vi "FlpLib ABCtoDQ_noSine_3PhasePowInv 4.vi"(0 "A":sgl, 1 "cosx":sgl, 2 "sinx":sgl, 5 "B":sgl, 7 "C":sgl) -> (4 "direct":sgl, 6 "quadrature":sgl, 10 "alpha":sgl, 15 "beta":sgl)   [LabVIEW 2017]
uses:
  ABCtoAlphaBeta_3PhasePowInv/FlpLib ABCtoAlphaBeta_3PhasePowInv 4.vi
  AlphaBetaToDQ_noSine/FlpLib AlphaBetaToDQ_noSine 4.vi
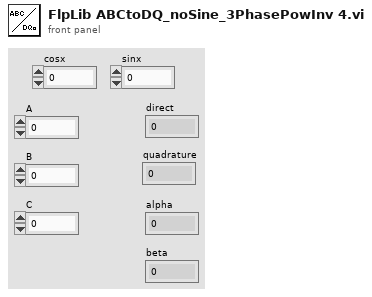
[diagram p1: front panel]
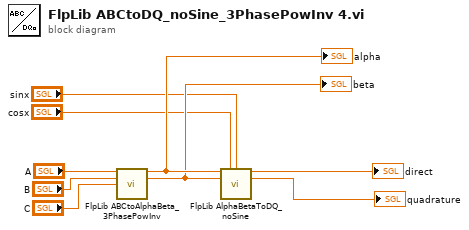
[diagram p0: block diagram]
diagram:
  n1 = call-poly "FlpLib ABCtoAlphaBeta_3PhasePowInv.vi"("A"="A", "B"="B", "C"="C") -> ("alpha"=w9:sgl, "beta"=w8:sgl)  [unwired: 11 in]
  "alpha" <- w9
  "beta" <- w8
  n2 = call-poly "FlpLib AlphaBetaToDQ_noSine.vi"("alpha"=w9, "cosx"="cosx", "sinx"="sinx", "beta"=w8) -> ("direct"=→"direct":sgl, "quadrature"=→"quadrature":sgl)  [unwired: 10 in]
